vi "Simulate_Keyboard.vi"(6 "error in (no error)":errorcluster, 8 "Action":u32(ring) items=["Down/Press", "Down then Up", "Up/Release"], 9 "Virtual Key":u8(ring) format="%.0x") -> (0 "error out":errorcluster)   [LabVIEW 2013]
uses:
  Windows/System32/user32.dll
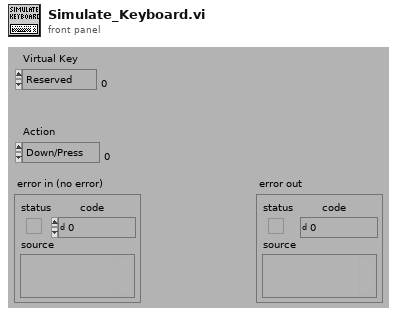
[diagram p1: front panel]
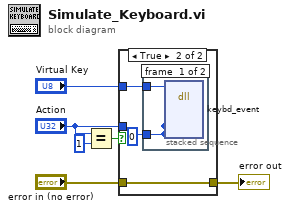
[diagram p0: block diagram]
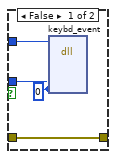
[diagram p2: hidden frame]
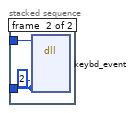
[diagram p3: hidden frame]
diagram:
  n1 = Equal?(x="Action", y=u32 1) -> (x = y?=w3:bool)
  n2 = case shown="True" w3 {
    tunnel: "Virtual Key" -> [w9 w13]
    tunnel: "Action" -> [w8 _]
    tunnel: [w7 w11] -> w1
    tunnel: "error in (no error)" -> [w7 w11]
    frame False {
      w10 = u32 0 ("dwFlags")
      n3 = dll-call lib="c:/Windows/System32/user32.dll" fn="keybd_event"("bVk"=w9, "bScan"=w10, "dwFlags"=w8, "dwExtraInfo"=w10) -> ()  [unwired: 8 in, 2 out]
    }
    frame True {
      n4 = stacked-sequence {
        tunnel: w13 -> [w15 w18]
        tunnel: u32 0 ("dwFlags") -> [w14 w17]
        frame #0 {
          n5 = dll-call lib="c:/Windows/System32/user32.dll" fn="keybd_event"("bVk"=w15, "bScan"=w14, "dwFlags"=w14, "dwExtraInfo"=w14) -> ()  [unwired: 8 in, 2 out]
        }
        frame #1 {
          n6 = dll-call lib="c:/Windows/System32/user32.dll" fn="keybd_event"("bVk"=w18, "bScan"=w17, "dwFlags"=u32 2, "dwExtraInfo"=w17) -> ()  [unwired: 8 in, 2 out]
        }
      }
    }
  }
  "error out" <- w1
